vi "disconnectTcpClientA.vi"(8 "error in (no error)":errorcluster, 10 "tel connection ID in":refnum<k5>, 11 "cmd connection ID in":refnum<k5>) -> (0 "error out":errorcluster)   [LabVIEW 2018]
doc: "Disconnect TCP server and TCP client, closing the TCP connection."
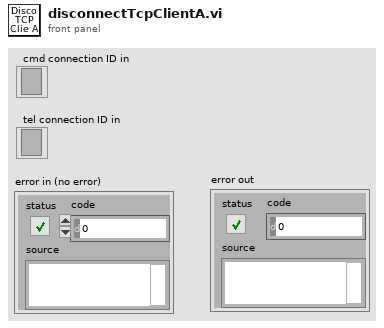
[diagram p1: front panel]
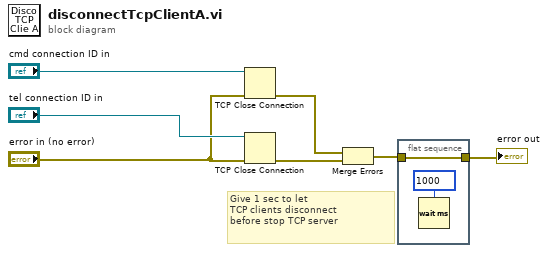
[diagram p0: block diagram]
diagram:
  # "Give 1 sec to let\nTCP clients disconnect\nbefore stop TCP server"
  n1 = TCP Close Connection(connection ID="cmd connection ID in", error in (no error)="error in (no error)") -> (error out=w5:errorcluster)  [unwired: 1 in, 1 out]
  n2 = TCP Close Connection(connection ID="tel connection ID in", error in (no error)="error in (no error)") -> (error out=w4:errorcluster)  [unwired: 1 in, 1 out]
  n3 = Merge Errors(w5, w4) -> (w2:errorcluster)
  n4 = flat-sequence {
    tunnel: w2 -> [w8]
    tunnel: [w8] -> w1
    frame #0 {
      n5 = Wait (ms)(milliseconds to wait=u32 1000) -> ()  [unwired: 1 out]
    }
  }
  "error out" <- w1
